vi "Write to File.vi"(8 "error in":errorcluster, 10 "File Actor In":refnum<class "File Actor.lvclass">, 11 "Exe Write Main in":refnum<class "Exe Write PAS Waveforms.lvclass">) -> (0 "error out":errorcluster, 2 "File Actor Out":refnum<class "File Actor.lvclass">)   [LabVIEW 2014, in "Controller.lvlib" / "Exe Write PAS Waveforms.lvclass"]
doc: "In this command, we pole the MAP DVR which contains all of the data that is to be written to file...."
uses:
  Exe Write PAS Waveforms.lvclass
  File Actor/File Actor.lvclass
  reusable/Data/Data.lvclass
  SuperActor/Ex Nested.lvclass/Ex Nested.ctl
  File Actor/File Actor.lvclass/File Actor.ctl
  Exe Write PAS Waveforms.lvclass/Exe Write PAS Waveforms.ctl
  reusable/PAS/Data/Main/PAS Data.lvclass
  SuperActor/Read Log Session.vi
  File Actor/Read File DVR.vi
  reusable/Data/Read measTime.vi
  reusable/PAS/Data/Main/Read CellData.vi
  reusable/PAS/Data/Cell/Read timeData.vi
  reusable/PAS/Data/Cell/Read lasDiodeData.vi
  <userlib>/_Session Fwk/Session - Root.lvclass
  reusable/PAS/Data/Cell/PAS Cell Data.lvclass
  reusable/Session APIs/Session Log/System Log.lvclass
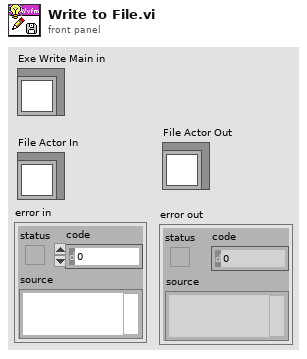
[diagram p1: front panel]
types:
  T1 = typedef "Session - Root.lvclass/Session Handle.ctl" = refnum<data-value>
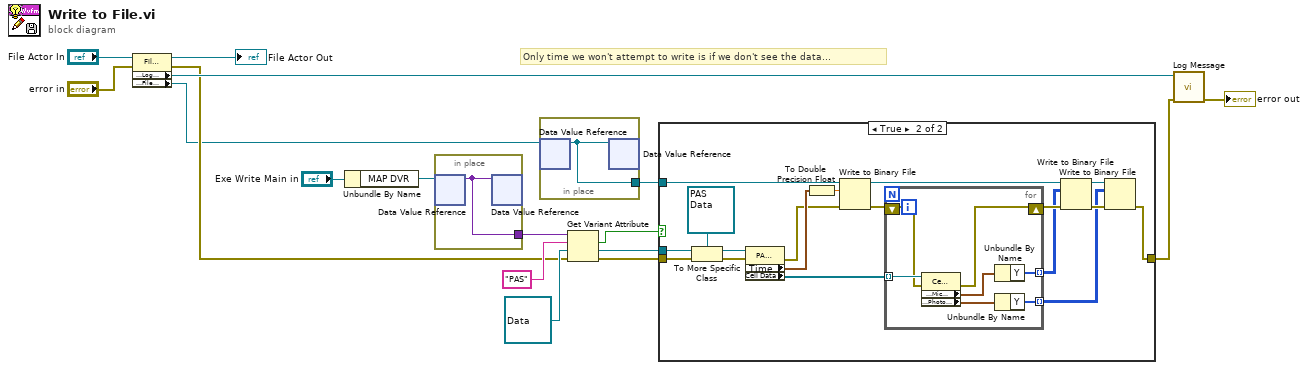
[diagram p0: block diagram]
diagram:
  # "Only time we won't attempt to write is if we don't see the data..."
  n1 = property class="File Actor"(reference="File Actor In", error in="error in") -> (reference out=→"File Actor Out":refnum<class "File Actor.lvclass">, error out=w2:errorcluster, "Accessors:Log Session"=w10:T1, "Accessors:File DVR"=w1:refnum<data-value>)
  n2 = Unbundle By Name("Exe Write Main in") -> ("MAP DVR"=w13:refnum<data-value>)
  n3 = in-place {
    in-place-border: [w18] -> w12
    n4 = in-place-dvr #1(w13) -> (w18:variant)  [unwired: 1 out]
    n5 = in-place-dvr #1(w18) -> ()  [unwired: 2 out]
  }
  n6 = in-place {
    in-place-border: [w19] -> w16
    n7 = in-place-dvr #2(w1) -> (w19:refnum<file>)  [unwired: 1 out]
    n8 = in-place-dvr #2(w19) -> ()  [unwired: 2 out]
  }
  n9 = Get Variant Attribute(Variant=w12, name="PAS", default value (empty Variant)=refnum<class "Data.lvclass"> refnum ("Base Data Lib:Data"), error in=w2) -> (found=w4:bool, value=w5:refnum<class "Data.lvclass">, error out=w3:errorcluster)  [unwired: 1 out]
  n10 = case shown="True" w4 {
    tunnel: [w20 w21] -> w9
    tunnel: w16 -> [_ w32]
    tunnel: w5 -> [_ w38]
    tunnel: w3 -> [w20 w30]
    frame False {
    }
    frame True {
      n11 = To More Specific Class(target class=refnum<class "PAS Data.lvclass"> refnum ("PAS Library.lvlib:PAS Data"), reference=w38, error in=w30) -> (specific class reference=w36:refnum<class "PAS Data.lvclass">, error out=w29:errorcluster)
      n12 = property class="PAS Data"(reference=w36, error in=w29) -> (error out=w28:errorcluster, "Time"=w34:timestamp, "Cell Data"=w35:refnum<class "PAS Cell Data.lvclass">[])  [unwired: 1 out]
      n13 = To Double Precision Float(number=w34) -> (double precision float=w33:dbl)
      n14 = Write to Binary File(file (use dialog)=w32, data=w33, error in=w28) -> (refnum out=w26:refnum<file>, error out=w31:errorcluster)  [unwired: 3 in, 1 out]
      n15 = for {
        tunnel: w35 -> [w45] mode=indexing
        shift-right: [w41] -> w27
        shift-left: w31 -> [w44]
        tunnel: [w40] -> w25 mode=indexing
        tunnel: [w39] -> w22 mode=indexing
        n16 = property class="Cell Data"(reference=w45, error in=w44) -> (error out=w41:errorcluster, "Accessors:Mic Time"=w43:waveform(i16), "Accessors:Photodiode"=w42:waveform(i16))  [unwired: 1 out]
        n17 = Unbundle By Name(w43) -> ("Y"=w40:i16[])
        n18 = Unbundle By Name(w42) -> ("Y"=w39:i16[])
      }
      n19 = Write to Binary File(file (use dialog)=w26, data=w25, error in=w27) -> (refnum out=w24:refnum<file>, error out=w23:errorcluster)  [unwired: 3 in, 1 out]
      n20 = Write to Binary File(file (use dialog)=w24, data=w22, error in=w23) -> (error out=w21:errorcluster)  [unwired: 3 in, 2 out]
    }
  }
  n21 = call "Log Message.vi"("error in"=w9, "session in"=w10) -> ("error out"=→"error out":errorcluster)  [unwired: 8 in, 1 out]
